vi "Is Reversing.vi"(10 "acceleration":dbl, 11 "velocity":dbl) -> (3 "Reversing?":bool)   [LabVIEW 2019]
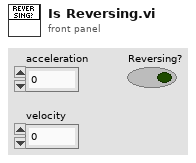
[diagram p1: front panel]
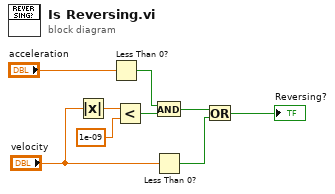
[diagram p0: block diagram]
diagram:
  n1 = Absolute Value(x="velocity") -> (abs(x)=w7:dbl)
  n2 = Less Than 0?(x="acceleration") -> (x < 0?=w3:bool)
  n3 = Less?(x=w7, y=1e-09) -> (x < y?=w5:bool)
  n4 = And(x=w3, y=w5) -> (x .and. y?=w2:bool)
  n5 = Less Than 0?(x="velocity") -> (x < 0?=w9:bool)
  n6 = Or(x=w2, y=w9) -> (x .or. y?=→"Reversing?":bool)
